vi "SetAvgTimes.vi"(2 "错误输入（无错误）":errorcluster, 3 "采样平均次数":u8) -> (0 "错误输出":errorcluster)   [LabVIEW 2018]
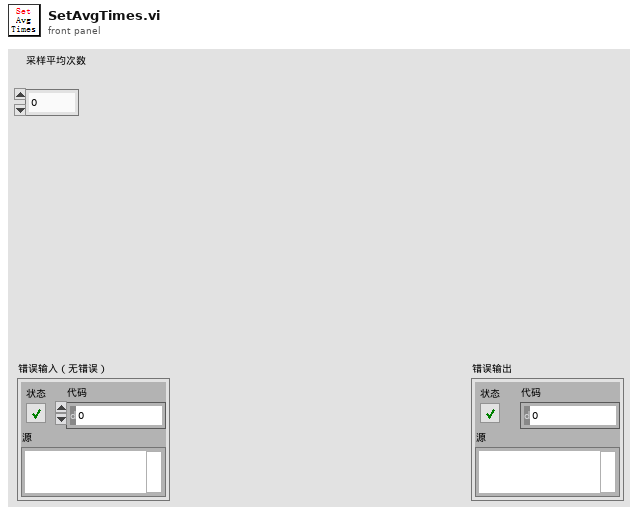
[diagram p1: front panel]
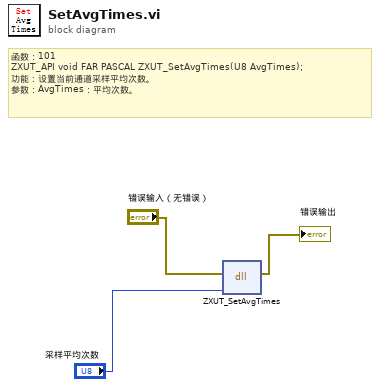
[diagram p0: block diagram]
diagram:
  # "函数：101\nZXUT_API void\tFAR PASCAL ZXUT_SetAvgTimes(U8 AvgTimes);\n功能：设置当前通道采样平均次数。\n参数：AvgTimes：平均次数。"
  n1 = dll-call lib="PTH2Rabs E软件项目超声超声子VI函数VI\tTCG处理ZXUTConfigMgr.dll" fn="ZXUT_SetAvgTimes"(error in="错误输入（无错误）", "AvgTimes"="采样平均次数") -> (error out=→"错误输出":errorcluster)  [unwired: 4 in, 1 out]
